vi "Do.vi"(6 "Input":variant, 8 "error in":errorcluster, 9 "Self Enqueuer":refnum<class "Message Enqueuer.lvclass">, 10 "Series Enqueuer":refnum<class "Message Enqueuer.lvclass">, 11 "Task Reply Time in":refnum<class "Task Reply Time.lvclass">) -> (0 "error out":errorcluster, 3 "Task Reply Time out":refnum<class "Task Reply Time.lvclass">)   [LabVIEW 2023, in "Task Reply Time.lvclass"]
uses:
  Task Reply Time.lvclass
  D:/git/HAL/HAL GOOP4/Task/Task Base/Task Base.lvclass
  <vilib>/ActorFramework/Message Enqueuer/Message Enqueuer.lvclass
  Task/Task Base/Task Base.lvclass/Task Base.ctl
  Task/ITask Actor/ITask Actor Messages/Do Msg/Do Msg.lvclass
  C:/Program Files/National Instruments/LabVIEW 2023/vi.lib/ActorFramework/Message/Message.lvclass
  gitlab/imponator-series-actor/Imponator Series Actor/Imponator Series UI Actor Messages/Log Event Msg/Log Event Msg.lvclass/Log Event Msg.ctl
  <vilib>/ActorFramework/Message Enqueuer/Message Enqueuer.lvclass/Message Enqueuer.ctl
  <vilib>/ActorFramework/Message Enqueuer/Enqueue.vi
  gitlab/imponator-series-actor/Imponator Series Actor/Imponator Series UI Actor Messages/Log Event Msg/Log Event Msg.lvclass
  <vilib>/Utility/LVClass/Get LV Class Name.vi
  <resource>/AFDebug/Generate Trace for Message.vi
  <vilib>/ActorFramework/Message Priority Queue/Priority Enqueue.vi
  Task Reply Time.lvclass/Task Reply Time.ctl
  Task/Task Base/Task Base.lvclass
  Measure and Stimulus Subsystems/Measure and Stimulus Subsystems.lvclass
  D:/git/HAL/HAL GOOP4/Tests/Sample Tasks/Test Reply Time/Task Reply Time.lvclass
  D:/git/HAL/HAL GOOP4/Task/ITask Actor/ITask Actor Messages/Do Msg/Do Msg.lvclass
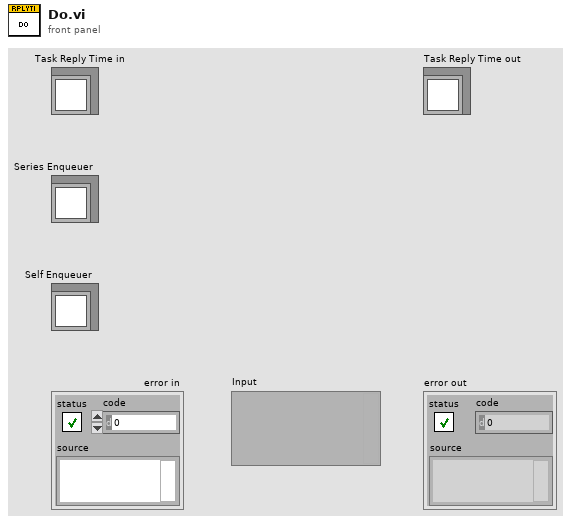
[diagram p1: front panel]
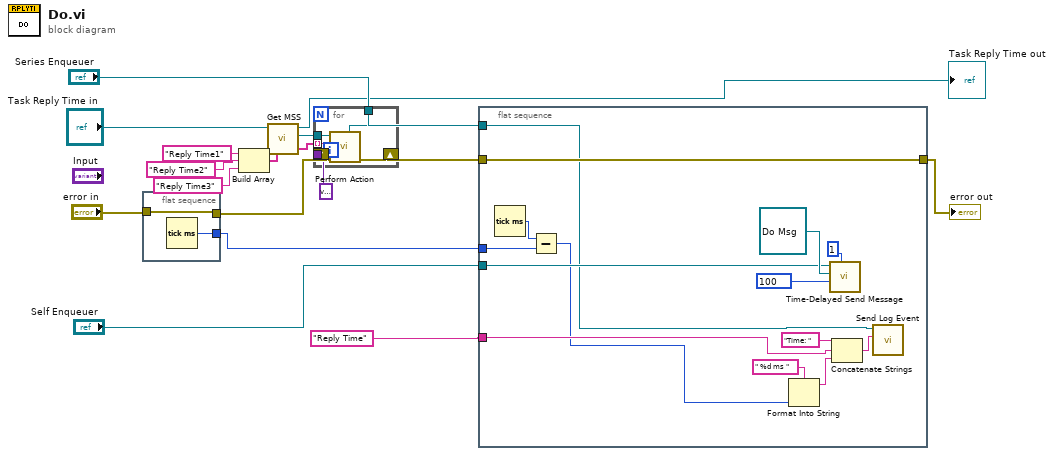
[diagram p0: block diagram]
diagram:
  n1 = flat-sequence {
    tunnel: "error in" -> [w18]
    tunnel: [w18] -> w13
    tunnel: [w17] -> w10
    frame #0 {
      n2 = Tick Count (ms)() -> (millisecond timer value=w17:u32)
    }
  }
  n3 = Build Array("Reply Time1" ("Point Ident"), "Reply Time2" ("Point Ident"), "Reply Time3" ("Point Ident")) -> (w1:string[])
  n4 = call "Get MSS.vi"("Task Base in"="Task Reply Time in") -> ("MSS"=w15:refnum<class "Measure and Stimulus Subsystems.lvclass">, "Task Base out"=→"Task Reply Time out":refnum<class "Task Reply Time.lvclass">)  [unwired: 9 in]
  n5 = for {
    tunnel: w15 -> [w24]
    tunnel: w1 -> [w23] mode=indexing
    tunnel: variant ("Input") -> [w21]
    tunnel: "Series Enqueuer" -> [w20]
    shift-right: [w19] -> w7
    shift-left: w13 -> [w22]
    n6 = call "Perform Action.vi"("Series Enqueuer"=w20, "error in"=w22, "Input"=w21, "Point Ident"=w23, "MSS in"=w24) -> ("error out"=w19:errorcluster)  [unwired: 3 in, 3 out]
  }
  n7 = flat-sequence {
    tunnel: w7 -> [w35]
    tunnel: "Self Enqueuer" -> [w33]
    tunnel: w10 -> [w36]
    tunnel: [w35] -> w6
    tunnel: "Reply Time" ("Ident") -> [w32]
    tunnel: "Series Enqueuer" -> [w30]
    frame #0 {
      n8 = Tick Count (ms)() -> (millisecond timer value=w37:u32)
      n9 = Subtract(x=w37, y=w36) -> (x-y=w29:u32)
      n10 = Format Into String(format string=" %d ms ", w29) -> (resulting string=w25:string)  [unwired: 2 in, 1 out]
      n11 = call <vilib>:"Time-Delayed Send Message.vi"("# Copies (0 = infinite repeat)"=u32 1, "Milliseconds To Wait"=100, "Message"=refnum<class "Do Msg.lvclass"> refnum ("HAL GOOP4.lvlib:ITask Actor.lvlib:Do Msg.lvclass"), "Message Enqueuer"=w33) -> ()  [unwired: 6 in, 2 out]
      n12 = Concatenate Strings("Time: " ("Event Text"), w32, w25) -> (w28:string)
      n13 = call "Send Log Event.vi"("Event Text"=w28, "Message Enqueuer"=w30) -> ()  [unwired: 8 in, 2 out]
    }
  }
  "error out" <- w6
